vi "Write target point.vi"(8 "error in (no error)":errorcluster, 10 "target point":cluster{"x":i16, "y":i16}, 11 "Target Point in":refnum<class "Target Point.lvclass">) -> (0 "error out":errorcluster, 3 "Target Point out":refnum<class "Target Point.lvclass">)   [LabVIEW 2014, in "Target Point.lvclass"]
uses:
  Target Point.lvclass
  Target Point.lvclass/Target Point.ctl
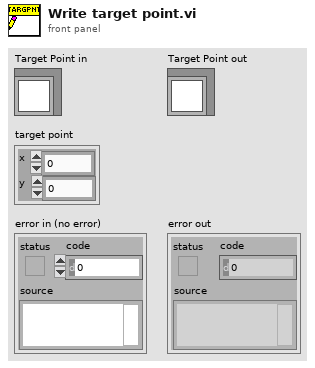
[diagram p1: front panel]
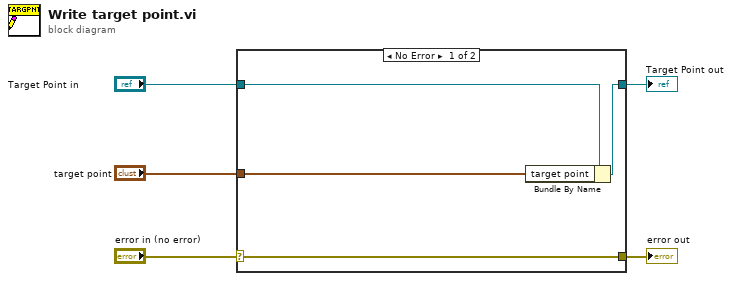
[diagram p0: block diagram]
diagram:
  n1 = case shown="No Error" "error in (no error)" {
    selector: "error in (no error)" -> [w9 w10]
    tunnel: [w9 w10] -> w4
    tunnel: [w7 w11] -> w2
    tunnel: "Target Point in" -> [w8 w11]
    tunnel: "target point" -> [w6 _]
    frame No Error {
      n2 = Bundle By Name(cluster=w8, "target point"=w6) -> (w7:refnum<class "Target Point.lvclass">)
    }
    frame Error {
    }
  }
  "error out" <- w4
  "Target Point out" <- w2
